vi "calibrate.vi"   [LabVIEW 2016]
uses:
  GLOBALS.vi
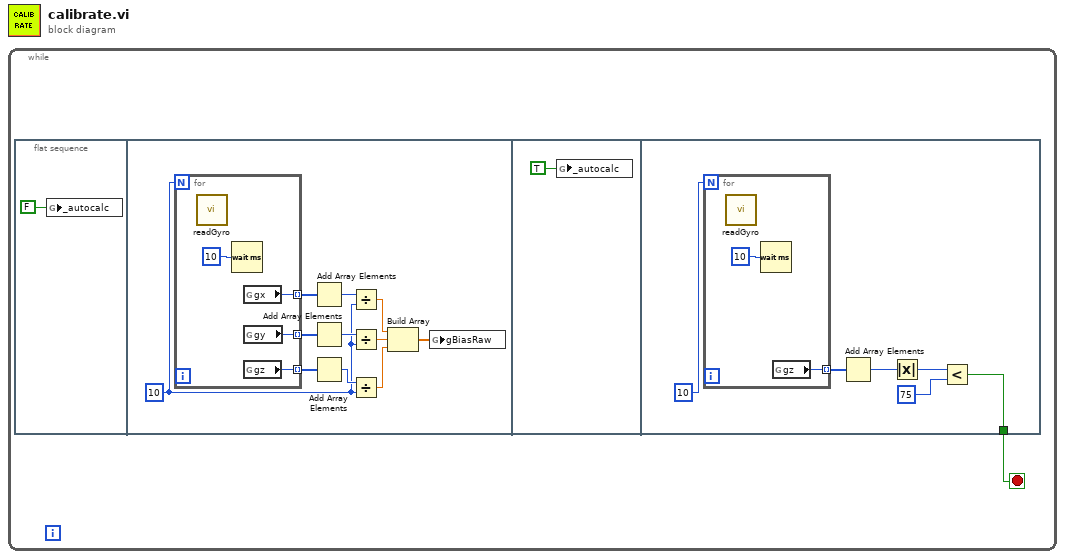
[diagram p0: block diagram]
diagram:
  n1 = while {
    stop <- w1 stop-if-true
    n2 = flat-sequence {
      tunnel: [w19] -> w1
      frame #0 {
        n3 = global write "GLOBALS.vi" "_autocalc"(FALSE ("_autocalc")) -> ()
      }
      frame #1 {
        w3 = u32 10 ("milliseconds to wait")
        n4 = for {
          N: w3 -> [_]
          tunnel: [w16] -> w13 mode=indexing
          tunnel: [w15] -> w12 mode=indexing
          tunnel: [w14] -> w11 mode=indexing
          n5 = call "readGyro.vi"() -> ()  [unwired: 12 in]
          n6 = Wait (ms)(milliseconds to wait=u32 10) -> ()  [unwired: 1 out]
          n7 = global read "GLOBALS.vi" "gx"() -> (w15:i16)
          n8 = global read "GLOBALS.vi" "gy"() -> (w16:i16)
          n9 = global read "GLOBALS.vi" "gz"() -> (w14:i16)
        }
        n10 = Add Array Elements(numeric array=w12) -> (sum=w8:i16)
        n11 = Add Array Elements(numeric array=w13) -> (sum=w10:i16)
        n12 = Add Array Elements(numeric array=w11) -> (sum=w9:i16)
        n13 = Divide(x=w8, y=w3) -> (x/y=w7:dbl)
        n14 = Divide(x=w10, y=w3) -> (x/y=w6:dbl)
        n15 = Divide(x=w9, y=w3) -> (x/y=w5:dbl)
        n16 = Build Array(w7, w6, w5) -> (w4:dbl[])
        n17 = global write "GLOBALS.vi" "gBiasRaw"(w4) -> ()
      }
      frame #2 {
        n18 = global write "GLOBALS.vi" "_autocalc"(TRUE ("_autocalc")) -> ()
      }
      frame #3 {
        n19 = for {
          N: u32 10 ("milliseconds to wait") -> [_]
          tunnel: [w25] -> w23 mode=indexing
          n20 = call "readGyro.vi"() -> ()  [unwired: 12 in]
          n21 = Wait (ms)(milliseconds to wait=u32 10) -> ()  [unwired: 1 out]
          n22 = global read "GLOBALS.vi" "gz"() -> (w25:i16)
        }
        n23 = Add Array Elements(numeric array=w23) -> (sum=w22:i16)
        n24 = Absolute Value(x=w22) -> (abs(x)=w21:i16)
        n25 = Less?(x=w21, y=i16 75) -> (x < y?=w19:bool)
      }
    }
  }
